vi "Set_predefined_table_positions.vi"(0 "Calibration IN":T2={"Calibration Y"=481893.0, "Calibration X"=487589.0} {"Calibration X" min=1.0 max=1000000.0; "Calibration Y" max=1000000.0}, 1 "Position Y":dbl=481445.0, 2 "Position X":dbl=481810.0, 5 "Reference IN":cluster{"Reference Y":dbl, "Reference X":dbl}={"Reference Y"=481816.0, "Reference X"=489241.0} {"Reference X" min=1.0 max=1000000.0; "Reference Y" max=1000000.0}, 9 "Centre IN":cluster{"Centre Y":dbl, "Centre X":dbl}={"Centre Y"=481816.0, "Centre X"=489241.0} {"Centre X" min=1.0 max=1000000.0; "Centre Y" max=1000000.0}, 11 "Park IN":T1={"Range Y"=250000.0, "Range X"=250000.0, "Range Z"=500000.0} {"Range Z" max=1000000.0; "Range X" min=1.0 max=1000000.0; "Range Y" max=1000000.0}) -> (4 "Calibration OUT":T2={"Calibration Y"=481893.0, "Calibration X"=487589.0} {"Calibration X" min=1.0 max=1000000.0; "Calibration Y" max=1000000.0}, 6 "Reference OUT":cluster{"Reference Y":dbl, "Reference X":dbl}={"Reference Y"=481810.0, "Reference X"=481445.0} {"Reference X" min=1.0 max=1000000.0; "Reference Y" max=1000000.0}, 10 "Centre OUT":cluster{"Centre Y":dbl, "Centre X":dbl}={"Centre Y"=481810.0, "Centre X"=481445.0} {"Centre X" min=1.0 max=1000000.0; "Centre Y" max=1000000.0}, 13 "Accept?":bool=TRUE, 15 "Park OUT":T1={"Range Y"=250000.0, "Range X"=250000.0, "Range Z"=500000.0} {"Range Z" max=1000000.0; "Range X" min=1.0 max=1000000.0; "Range Y" max=1000000.0})   [LabVIEW 2011]
panel:
  in  "undo":bool
  in  "accept":bool
  in  "Rangement Z":dbl=500000.0 min=-1000000.0 max=1000000.0
  in  "copy_calib":bool
  in  "copy_ref":bool
  in  "copy_centre":bool
  in  "Calibration X":dbl=481893.0 min=1.0 max=1000000.0
  in  "Calibration Y":dbl=487589.0 max=1000000.0
  in  "Reference X":dbl=481810.0 min=0.0 max=1000000.0
  in  "Reference Y":dbl=481445.0 min=0.0 max=1000000.0
  in  "CentreRot X":dbl=481810.0 min=1.0 max=1000000.0
  in  "CentreRot Y":dbl=481445.0 max=1000000.0
  in  "Rangement X":dbl=250000.0 min=-1000000.0 max=1000000.0
  in  "Rangement Y":dbl=250000.0 min=-1000000.0 max=1000000.0
  # "La position de calibration est la position pour laquelle \nle miroir de calibration devrait se retrouver face au lampe"
  # "La position de référence est celle pour laquelle le centre de la caméra de guidage correspond à la coordonnée synchronisée du télescope"
  # "Le centre de rotation est la position autour de laquelle\nla bonnette tourne.  Si vous travailler à des angles autres que  0°, il est essentiel que cette coordonnées soit bonne."
  # "La position de rangement est celle à laquelle il est recommandé de positionner les tables de translation\nlors de l'arrêt du système."
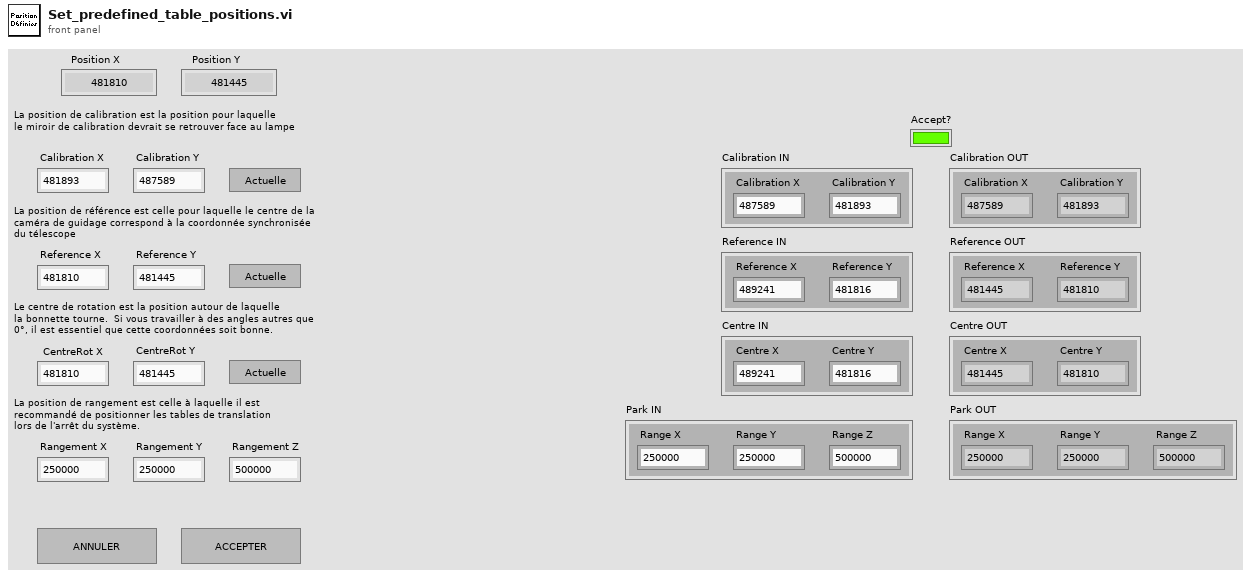
[diagram p1: front panel]
types:
  T1 = cluster{"Range Y":dbl, "Range X":dbl, "Range Z":dbl}
  T2 = cluster{"Calibration Y":dbl, "Calibration X":dbl}
  T3 = cluster{"Calibration X":dbl, "Calibration Y":dbl}
  T4 = cluster{"Rangement X":dbl, "Rangement Y":dbl, "Rangement Z":dbl}
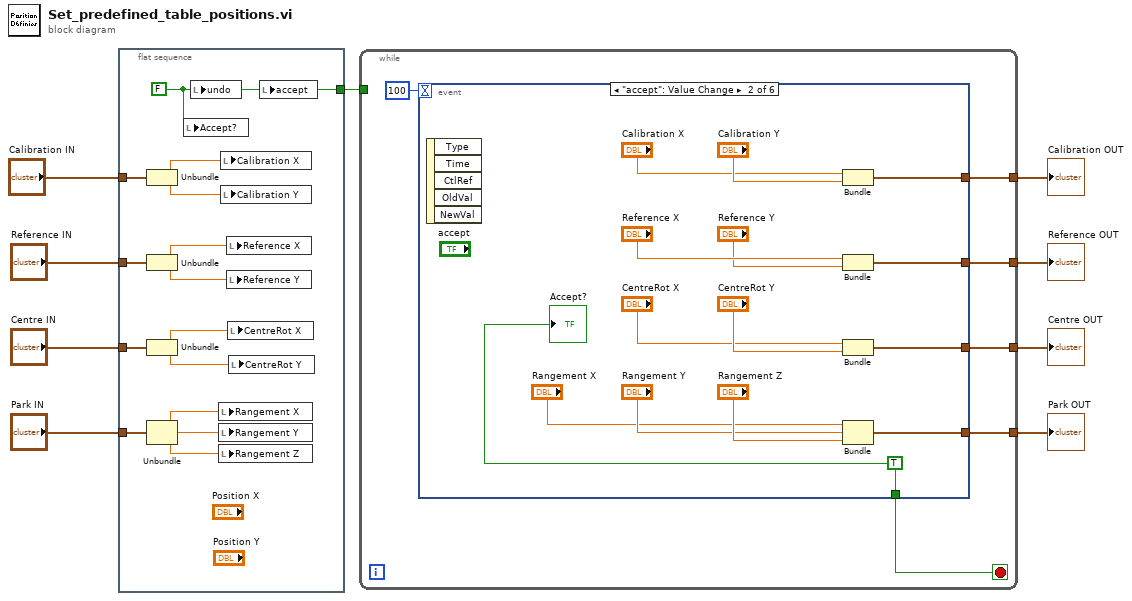
[diagram p0: block diagram]
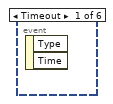
[diagram p2: hidden frame]
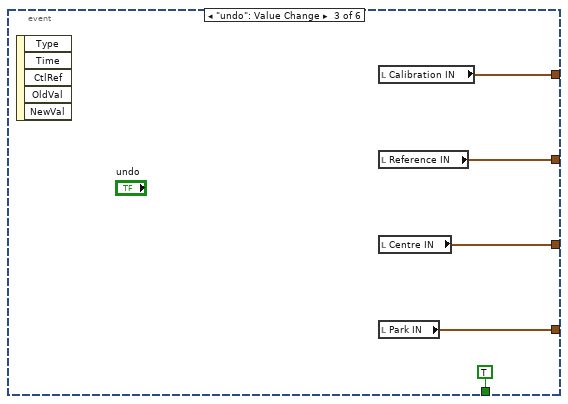
[diagram p3: hidden frame]
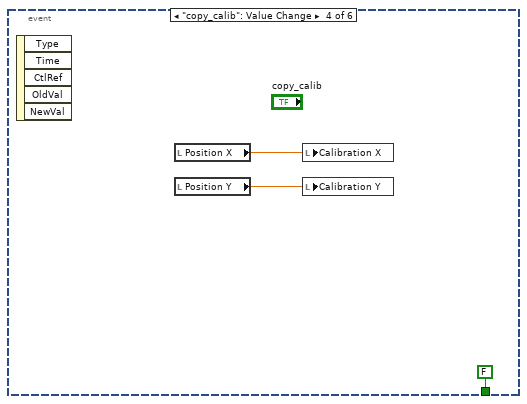
[diagram p4: hidden frame]
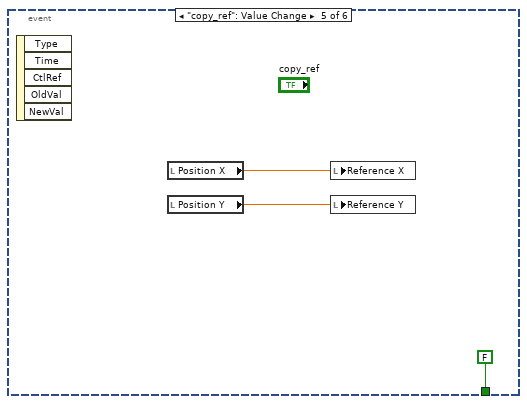
[diagram p5: hidden frame]
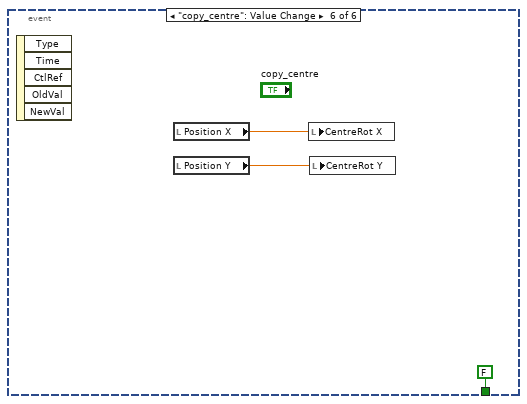
[diagram p6: hidden frame]
diagram:
  n1 = flat-sequence {
    tunnel: "Calibration IN" -> [w23]
    tunnel: "Reference IN" -> [w16]
    tunnel: "Centre IN" -> [w17]
    tunnel: "Park IN" -> [w15]
    tunnel: [w10] -> w5
    frame #0 {
      w10 = FALSE
      n2 = Unbundle(w23) -> ("Calibration Y"=w11:dbl, "Calibration X"=w22:dbl)
      n3 = Unbundle(w16) -> ("Reference Y"=w20:dbl, "Reference X"=w21:dbl)
      n4 = Unbundle(w17) -> ("Centre Y"=w19:dbl, "Centre X"=w18:dbl)
      n5 = Unbundle(w15) -> ("Range Y"=w14:dbl, "Range X"=w12:dbl, "Range Z"=w13:dbl)
      n6 = local write "Accept?"(w10) -> ()
      n7 = local write "undo"(w10) -> ()
      n8 = local write "Rangement X"(w14) -> ()
      n9 = local write "Rangement Y"(w12) -> ()
      n10 = local write "Rangement Z"(w13) -> ()
      n11 = local write "Calibration X"(w11) -> ()
      n12 = local write "Calibration Y"(w22) -> ()
      n13 = local write "Reference X"(w20) -> ()
      n14 = local write "Reference Y"(w21) -> ()
      n15 = local write "CentreRot X"(w19) -> ()
      n16 = local write "CentreRot Y"(w18) -> ()
      n17 = local write "accept"(w10) -> ()
    }
  }
  n18 = while {
    tunnel: w5 -> [_]
    tunnel: [w28] -> w4
    tunnel: [w27] -> w3
    tunnel: [w26] -> w2
    tunnel: [w25] -> w1
    stop <- w24 stop-if-true
    n19 = event shown="[1] \"accept\": Value Change" {
      selector: _ -> [_ _ _ _ _ _]
      dyn-events: _ -> [_ _ _ _ _ _]
      timeout: 100 -> [_ _ _ _ _ _]
      tunnel: [_ w40 w48 _ _ _] -> w28
      tunnel: [_ w39 w47 _ _ _] -> w27
      tunnel: [_ w38 w46 _ _ _] -> w26
      tunnel: [_ w43 w45 _ _ _] -> w25
      tunnel: [_ w30 TRUE FALSE FALSE FALSE] -> w24
      event Timeout {
        n20 = event-data() -> ()  [unwired: 1 in, 2 out]
      }
      event "accept": Value Change {
        w30 = TRUE
        n21 = event-data() -> ()  [unwired: 1 in, 5 out]
        n22 = Bundle("Calibration X"="Calibration X", "Calibration Y"="Calibration Y") -> (w43:T3)  [unwired: 1 in]
        n23 = Bundle("Reference X"="Reference X", "Reference Y"="Reference Y") -> (w38:cluster{"Reference X":dbl, "Reference Y":dbl})  [unwired: 1 in]
        n24 = Bundle("CentreRot X"="CentreRot X", "CentreRot Y"="CentreRot Y") -> (w39:cluster{"CentreRot X":dbl, "CentreRot Y":dbl})  [unwired: 1 in]
        n25 = Bundle("Rangement X"="Rangement X", "Rangement Y"="Rangement Y", "Rangement Z"="Rangement Z") -> (w40:T4)  [unwired: 1 in]
        "Accept?" <- w30
      }
      event "undo": Value Change {
        n26 = event-data() -> ()  [unwired: 1 in, 5 out]
        n27 = local read "Calibration IN"() -> (w45:T2)
        n28 = local read "Reference IN"() -> (w46:cluster{"Reference Y":dbl, "Reference X":dbl})
        n29 = local read "Centre IN"() -> (w47:cluster{"Centre Y":dbl, "Centre X":dbl})
        n30 = local read "Park IN"() -> (w48:T1)
      }
      event "copy_calib": Value Change {
        n31 = event-data() -> ()  [unwired: 1 in, 5 out]
        n32 = local read "Position X"() -> (w51:dbl)
        n33 = local read "Position Y"() -> (w50:dbl)
        n34 = local write "Calibration X"(w51) -> ()
        n35 = local write "Calibration Y"(w50) -> ()
      }
      event "copy_ref": Value Change {
        n36 = event-data() -> ()  [unwired: 1 in, 5 out]
        n37 = local read "Position X"() -> (w54:dbl)
        n38 = local read "Position Y"() -> (w53:dbl)
        n39 = local write "Reference X"(w54) -> ()
        n40 = local write "Reference Y"(w53) -> ()
      }
      event "copy_centre": Value Change {
        n41 = event-data() -> ()  [unwired: 1 in, 5 out]
        n42 = local read "Position X"() -> (w57:dbl)
        n43 = local read "Position Y"() -> (w56:dbl)
        n44 = local write "CentreRot X"(w57) -> ()
        n45 = local write "CentreRot Y"(w56) -> ()
      }
    }
  }
  "Calibration OUT" <- w1
  "Reference OUT" <- w2
  "Centre OUT" <- w3
  "Park OUT" <- w4
